vi "Current Sense card.vi"(8 "error in (no error)":errorcluster, 11 "Node Ptr":T4 format="%.0x") -> (0 "error out":errorcluster)   [LabVIEW 2014, in "SLSC configuration System Explorer.lvlib"]
uses:
  SLSC configuration System Explorer.lvlib
  <vilib>/NI Veristand/Custom Device API/Custom Device Item Ref.ctl
  Type Defs/Card Position.ctl
  Shared/SPI Utility/Slot #.ctl
  Shared/Current Sense Board/Current Sense Calibration State.ctl
  <vilib>/NI Veristand/Custom Device API/Custom Device API.lvlib
  Shared/SLSC configuration Shared.lvlib
panel:
  in  "Calibration State Initial Value":T1
  in  "Card Position":T2 {"Slot #" max=15}
  in  "Header 2":cluster{"Section Name":string}={"Section Name"="Bank 0 Settings"}
  in  "Header":cluster{"Section Name":string}={"Section Name"="Current Sense Card Settings"}
  in  "Description":string
  in  "Name":string
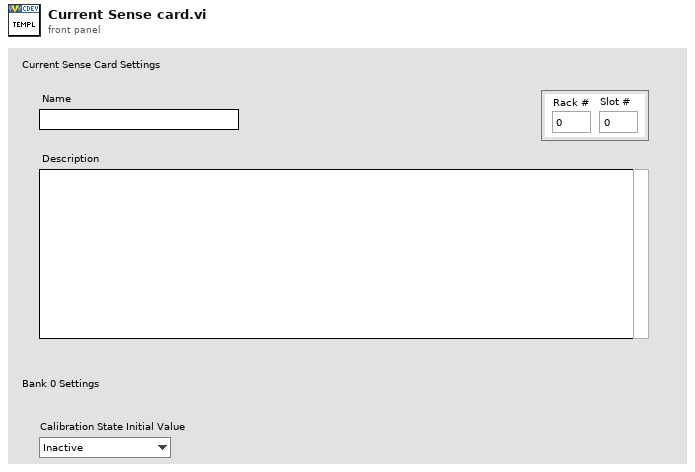
[diagram p1: front panel]
types:
  T1 = typedef "SLSC configuration Shared.lvlib/Current Sense Calibration State.ctl" = enum16{"Inactive", "Channel 1", "Channel 2", "Channel 3", "Channel 4", "Channel 5", "Channel 6", "Channel 7", "Channel 8", "Channel 9", "Channel 10", "Channel 11", "Channel 12", "Channel 13", "Channel 14", "Channel 15", "Channel 16"}
  T2 = typedef "SLSC configuration Shared.lvlib/Card Position.ctl" = cluster{"Rack #":u8, "Slot #":T3}
  T3 = typedef "SLSC configuration Shared.lvlib/Slot #.ctl" = u8
  T4 = typedef "Custom Device API.lvlib/Custom Device Item Ref.ctl" = u64
  T5 = typedef "Custom Device API.lvlib/Custom Device Item Info.ctl" = cluster{"Name":string, "Is Channel":bool, "GUID":string, "Is Waveform":bool}
  T6 = typedef "Custom Device API.lvlib/Custom Device Commands.ctl" = enum16{"Default", "Item renamed", "Shutdown", "Dynamic button pressed"}
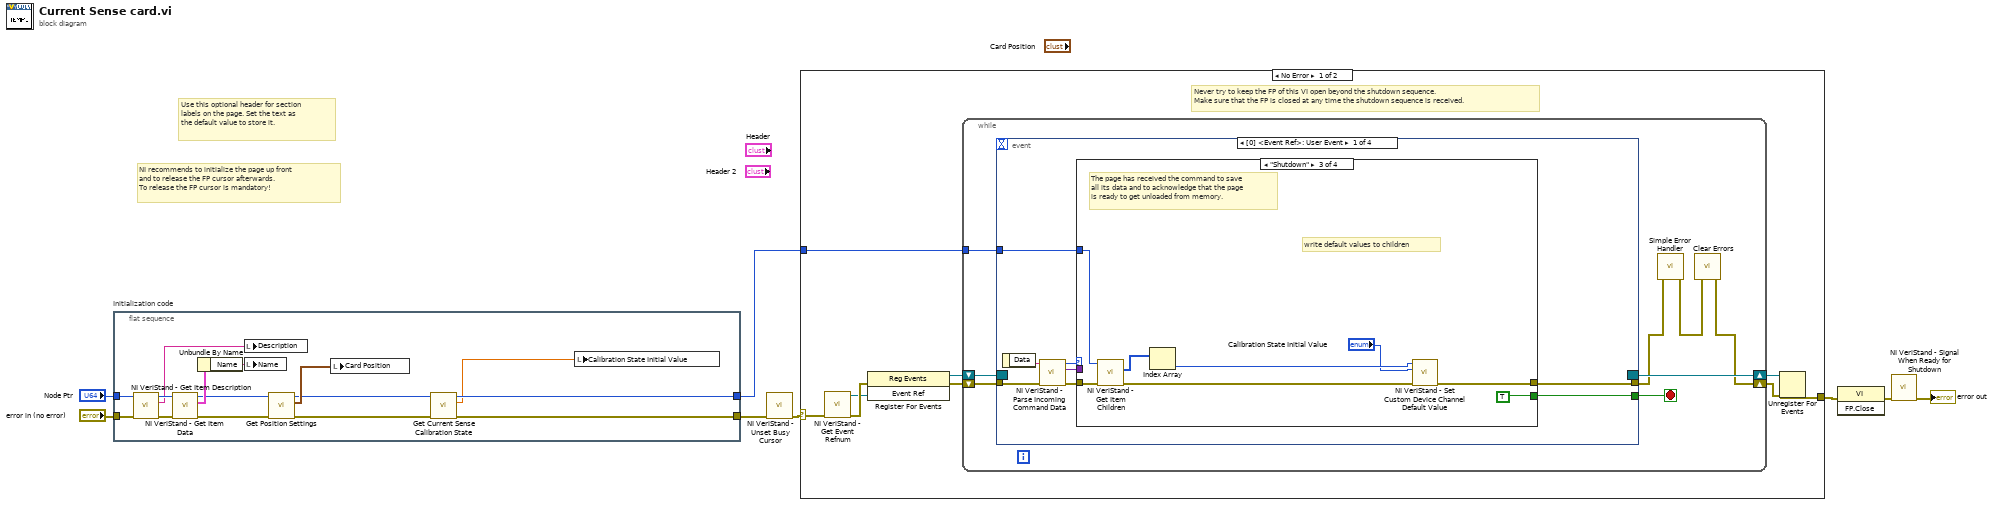
[diagram p0: block diagram]
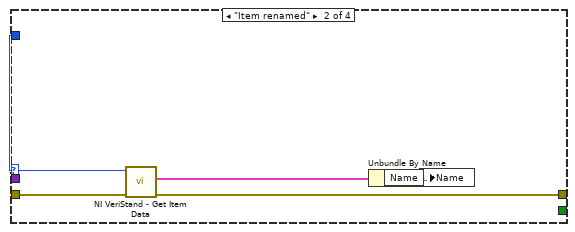
[diagram p3: hidden frame]
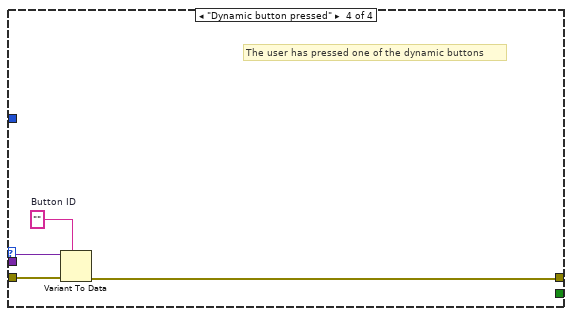
[diagram p4: hidden frame]
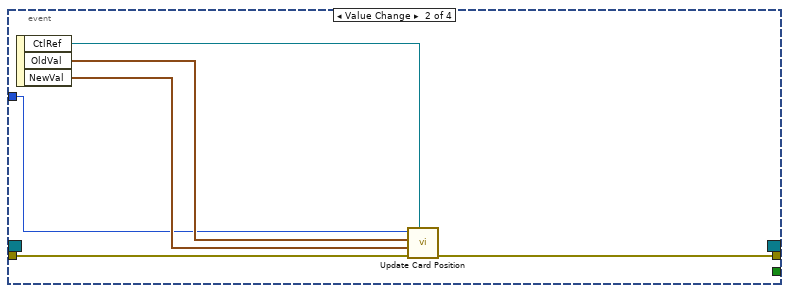
[diagram p5: hidden frame]
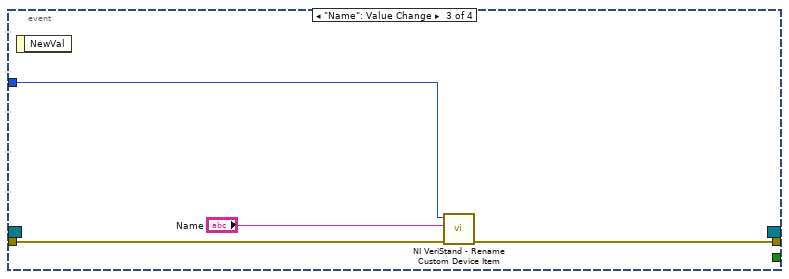
[diagram p6: hidden frame]
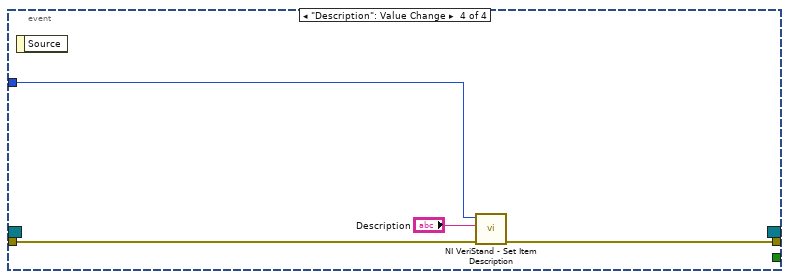
[diagram p7: hidden frame]
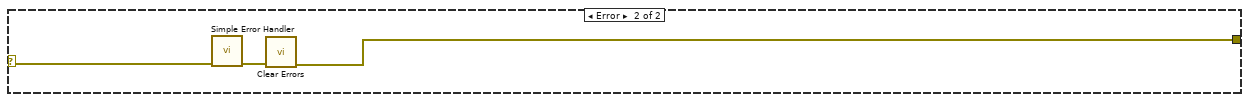
[diagram p8: hidden frame]
diagram:
  # "Use this optional header for section labels on the page. Set the text as the default value to store it."
  # "NI recommends to initialize the page up front\nand to release the FP cursor afterwards.\nTo release the FP cursor is mandatory!"
  n1 = flat-sequence "Initialization code" {
    tunnel: "error in (no error)" -> [w22]
    tunnel: "Node Ptr" -> [w21]
    tunnel: [w11] -> w4
    tunnel: [w10] -> w1
    frame #0 {
      n2 = call <vilib>:"NI VeriStand - Get Item Description.vi"("error in (no error)"=w22, "Item Ref in"=w21) -> ("error out"=w19:errorcluster, "Description"=w20:string, "Item Ref out"=w23:T4)  [unwired: 7 out]
      n3 = call <vilib>:"NI VeriStand - Get Item Data.vi"("error in (no error)"=w19, "Item Ref in"=w23) -> ("error out"=w16:errorcluster, "Item Info"=w18:T5, "Item Ref out"=w15:T4)  [unwired: 7 out]
      n4 = Unbundle By Name(w18) -> ("Name"=w17:string)
      n5 = local write "Description"(w20) -> ()
      n6 = local write "Name"(w17) -> ()
      n7 = call "Get Position Settings.vi"("error in (no error)"=w16, "Item Ref in"=w15) -> ("error out"=w12:errorcluster, "Card Position"=w14:T2, "Item Ref out"=w13:T4)  [unwired: 7 in]
      n8 = local write "Card Position"(w14) -> ()
      n9 = call "Get Current Sense Calibration State.vi"("error in (no error)"=w12, "Item Ref in"=w13) -> ("error out"=w11:errorcluster, "Calibration State"=w9:dbl, "Item Ref out"=w10:T4)  [unwired: 6 in, 1 out]
      n10 = local write "Calibration State Initial Value"(w9) -> ()
    }
  }
  n11 = call <vilib>:"NI VeriStand - Unset Busy Cursor.vi"("error in (no error)"=w4) -> ("error out"=w3:errorcluster)  [unwired: 10 out]
  n12 = case shown="No Error" w3 {
    selector: w3 -> [w24 w83]
    tunnel: [w29 w81] -> w8
    tunnel: w1 -> [w25 _]
    frame No Error {
      # "Never try to keep the FP of this VI open beyond the shutdown sequence.\nMake sure that the FP is closed at any time the shutdown sequence is received."
      n13 = call <vilib>:"NI VeriStand - Get Event Refnum.vi"("error in (no error)"=w24) -> ("error out"=w32:errorcluster, "Event Ref"=w28:refnum<user-event>)  [unwired: 9 out]
      n14 = register-events(error in=w32, w28) -> (reference out=w26:refnum<event-registration>, error out=w27:errorcluster)  [unwired: 1 in]
      n15 = while {
        tunnel: w25 -> [w36]
        shift-right: [w33] -> w30
        shift-left: w27 -> [w39]
        shift-right: [w40] -> w31
        shift-left: w26 -> [w38]
        stop <- w37 stop-if-true
        n16 = event shown="[0] <Event Ref>: User Event" {
          selector: w38 -> [_ _ _ _]
          dyn-events: [_ _ _ _] -> w40
          timeout: _ -> [_ _ _ _]
          tunnel: w39 -> [w48 w72 w76 w79]
          tunnel: [w44 _ _ _] -> w37
          tunnel: [w43 w71 w75 w78] -> w35
          tunnel: w36 -> [w42 w68 w74 w80]
          event User Event {
            n17 = event-data() -> ("Data"=w47:string)  [unwired: 1 out]
            n18 = call <vilib>:"NI VeriStand - Parse Incoming Command Data.vi"("error in (no error)"=w48, "Incoming data"=w47) -> ("error out"=w46:errorcluster, "Outgoing data"=w41:variant, "Action"=w45:T6)  [unwired: 7 out]
            n19 = case shown="\"Shutdown\"" w45 {
              tunnel: w46 -> [w49 w54 w61 w66]
              tunnel: [_ _ TRUE _] -> w44
              tunnel: [w49 w51 w59 w63] -> w43
              tunnel: w42 -> [_ w53 w60 _]
              tunnel: w41 -> [_ _ _ w65]
              frame "Default", Default {
              }
              frame "Item renamed" {
                n20 = call <vilib>:"NI VeriStand - Get Item Data.vi"("error in (no error)"=w54, "Item Ref in"=w53) -> ("error out"=w51:errorcluster, "Item Info"=w52:T5)  [unwired: 8 out]
                n21 = Unbundle By Name(w52) -> ("Name"=w50:string)
                n22 = local write "Name"(w50) -> ()
              }
              frame "Shutdown" {
                # "write default values to children"
                # "The page has received the command to save all its data and to acknowledge that the page is ready to get unloaded from memory."
                n23 = call <vilib>:"NI VeriStand - Get Item Children.vi"("error in (no error)"=w61, "Item Ref in"=w60) -> ("error out"=w57:errorcluster, "Child Refs"=w58:T4[])  [unwired: 6 in, 2 out]
                n24 = Index Array(array=w58) -> (element=w56:T4)  [unwired: 1 in]
                n25 = call <vilib>:"NI VeriStand - Set Custom Device Channel Default Value.vi"("error in (no error)"=w57, "Default Value"="Calibration State Initial Value", "Channel Ref in"=w56) -> ("error out"=w59:errorcluster)  [unwired: 7 in, 1 out]
              }
              frame "Dynamic button pressed" {
                w64 = ""  # Button ID
                # "The user has pressed one of the dynamic buttons"
                n26 = Variant To Data(error in=w66, type=w64, Variant=w65) -> (error out=w63:errorcluster)  [unwired: 1 out]
              }
            }
          }
          event Value Change {
            n27 = event-data() -> ("CtlRef"=w67:refnum<vi>, "OldVal"=w69:T2, "NewVal"=w70:T2)  [unwired: 1 out]
            n28 = call "Update Card Position.vi"("Card Position Ref"=w67, "error in (no error)"=w72, "NewVal"=w70, "OldVal"=w69, "Node Ptr in"=w68) -> ("error out"=w71:errorcluster)  [unwired: 6 in]
          }
          event "Name": Value Change {
            n29 = event-data() -> ()  [unwired: 2 out]
            n30 = call <vilib>:"NI VeriStand - Rename Custom Device Item.vi"("error in (no error)"=w76, "New Name"="Name", "Item Ref in"=w74) -> ("error out"=w75:errorcluster)  [unwired: 1 in, 7 out]
          }
          event "Description": Value Change {
            n31 = event-data() -> ()  [unwired: 2 out]
            n32 = call <vilib>:"NI VeriStand - Set Item Description.vi"("error in (no error)"=w79, "Description"="Description", "Item Ref in"=w80) -> ("error out"=w78:errorcluster)  [unwired: 8 out]
          }
        }
        n33 = call <vilib>:"Simple Error Handler.vi"("error in (no error)"=w35) -> ("error out"=w34:errorcluster)  [unwired: 1 in, 7 out]
        n34 = call <vilib>:"Clear Errors.vi"("error in (no error)"=w34) -> ("error out"=w33:errorcluster)  [unwired: 1 in, 5 out]
      }
      n35 = Unregister For Events(event registration refnum=w31, error in=w30) -> (error out=w29:errorcluster)
    }
    frame Error {
      n36 = call <vilib>:"Simple Error Handler.vi"("error in (no error)"=w83) -> ("error out"=w82:errorcluster)  [unwired: 1 in, 7 out]
      n37 = call <vilib>:"Clear Errors.vi"("error in (no error)"=w82) -> ("error out"=w81:errorcluster)  [unwired: 1 in, 5 out]
    }
  }
  n38 = invoke class="VI" method="FP.Close"(error in=w8) -> (error out=w7:errorcluster)  [unwired: 2 in, 2 out]
  n39 = call <vilib>:"NI VeriStand - Signal When Ready for Shutdown.vi"("error in (no error)"=w7) -> ("error out"=→"error out":errorcluster)  [unwired: 10 out]
